vi "BuildAccessorFunctions.vi"(8 "error in (no error)":errorcluster, 11 "CS++Actor in":refnum<class "CS++Actor.lvclass">) -> (0 "error out":errorcluster, 3 "CS++Actor out":refnum<class "CS++Actor.lvclass">)   [LabVIEW 2016, in "CS++Actor.lvlib" / "CS++Actor.lvclass"]
uses:
  CS++Actor.lvclass
  CS++Actor.lvclass/CS++Actor.ctl
  <vilib>/Utility/traverseref.llb/TRef TravTarget.ctl
  <resource>/Framework/Providers/LVClassLibrary/NewAccessors/MemberVICreation.lvlib
  <vilib>/Utility/traverseref.llb/VI Scripting - Traverse.lvlib
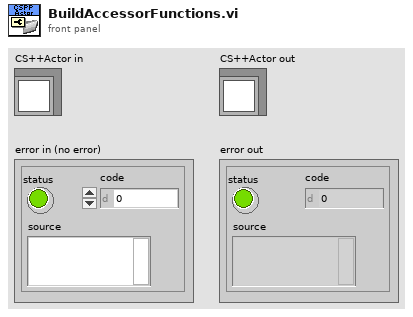
[diagram p1: front panel]
types:
  T1 = typedef "TRef TravTarget.ctl" = enum16{"FP", "BD", "Other"}
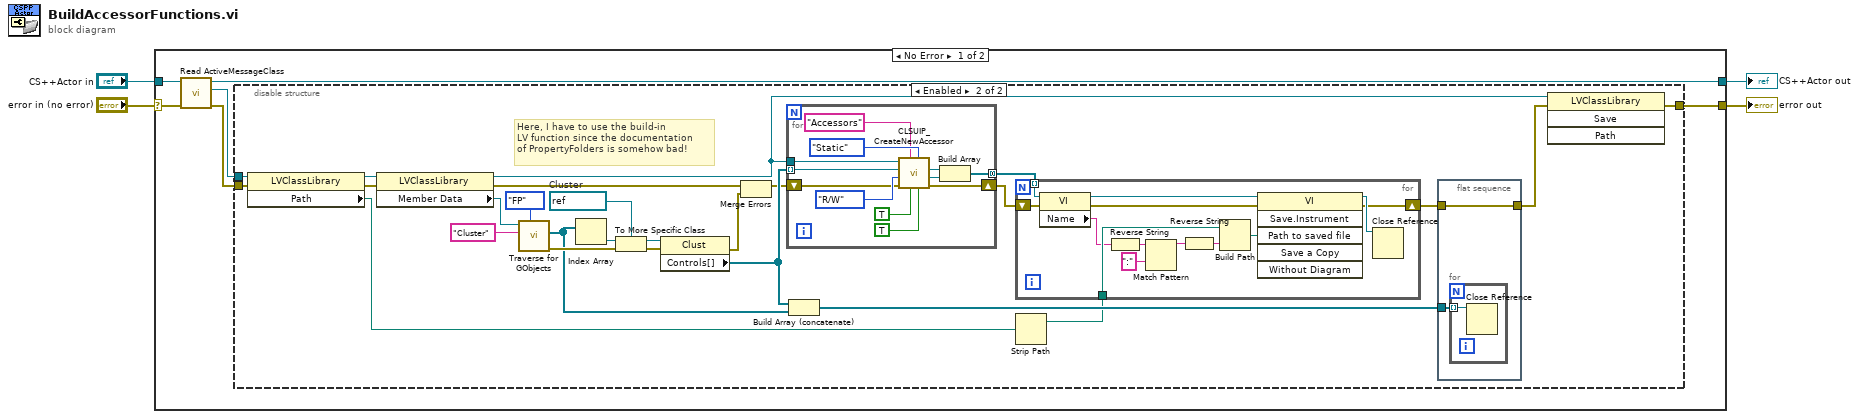
[diagram p0: block diagram]
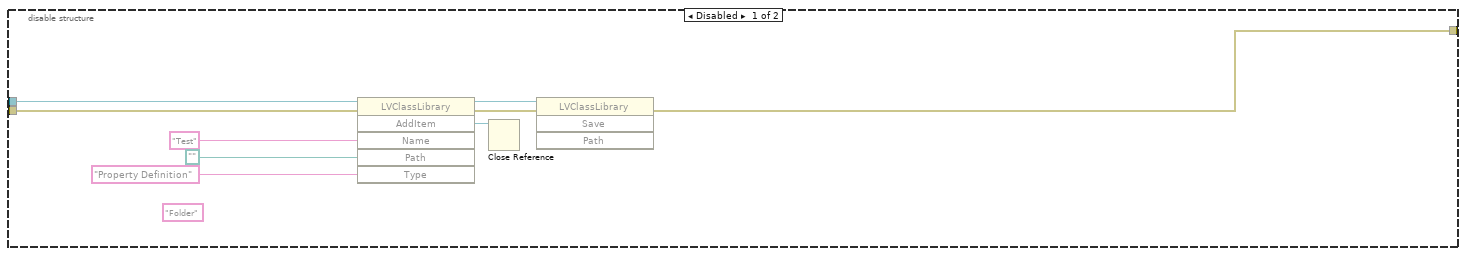
[diagram p2: hidden frame]
diagram:
  n1 = case shown="No Error" "error in (no error)" {
    selector: "error in (no error)" -> [w8 w75]
    tunnel: [w5 w75] -> w3
    tunnel: [w9 w74] -> w1
    tunnel: "CS++Actor in" -> [w10 w74]
    frame No Error {
      n2 = call "Read ActiveMessageClass.vi"("error in (no error)"=w8, "CS++Actor in"=w10) -> ("error out"=w6:errorcluster, "ActiveMessageClass"=w7:refnum<vi>, "CS++Actor out"=w9:refnum<class "CS++Actor.lvclass">)  [unwired: 7 in]
      n3 = disable-structure shown="Enabled" {
        disable-tunnel: w7 -> [w19 w29]
        disable-tunnel: w6 -> [w18 w27]
        disable-tunnel: [w12 w35] -> w5
        frame Disabled {
          (unwired) "Folder" ("Type")
          n4 = invoke class="LVClassLibrary" method="AddItem"(reference=w19, error in=w18, "Name"="Test" ("Type"), "Path"=path "", "Type"="Property Definition") -> (reference out=w14:refnum<vi>, error out=w13:errorcluster, "AddItem"=w15:refnum<vi>)  [unwired: 1 in, 3 out]
          n5 = Close Reference(reference=w15) -> ()  [unwired: 1 in, 1 out]
          n6 = invoke class="LVClassLibrary" method="Save"(reference=w14, error in=w13) -> (error out=w12:errorcluster)  [unwired: 2 in, 3 out]
        }
        frame Enabled {
          w42 = refnum<vi> refnum  # Cluster
          # "Here, I have to use the build-in\nLV function since the documentation\nof PropertyFolders is somehow bad!"
          n7 = property class="LVClassLibrary"(reference=w29, error in=w27) -> (reference out=w28:refnum<vi>, error out=w26:errorcluster, "Path"=w25:path)
          n8 = property class="LVClassLibrary"(reference=w28, error in=w26) -> (reference out=w33:refnum<vi>, error out=w22:errorcluster, "Member Data"=w38:refnum<vi>)
          n9 = call <vilib>:"Traverse for GObjects.vi"("Traverse Target"=TRef_TravTarget."FP", "Class Name"="Cluster" ("name/order"), "VI Refnum"=w38) -> ("error out"=w41:errorcluster, "References"=w36:refnum<vi>[])  [unwired: 5 in, 2 out]
          n10 = Index Array(array=w36) -> (element=w43:refnum<vi>)  [unwired: 1 in]
          n11 = To More Specific Class(target class=w42, reference=w43, error in=w41) -> (specific class reference=w39:refnum<vi>, error out=w40:errorcluster)
          n12 = property class="Clust"(reference=w39, error in=w40) -> (error out=w21:errorcluster, "Controls[]"=w23:refnum<vi>[])  [unwired: 1 out]
          n13 = Merge Errors(w22, w21) -> (w20:errorcluster)
          n14 = for {
            tunnel: w23 -> [w54] mode=indexing
            tunnel: w33 -> [w53]
            tunnel: [w50] -> w32 mode=concatenating
            shift-right: [w49] -> w31
            shift-left: w20 -> [w55]
            n15 = call <resource>:"CLSUIP_CreateNewAccessor.vi"("Make available through Property Nodes"=TRUE, "VI Type"=enum32{"Dynamic", "Static"}."Static", "Include error terminals"=TRUE, "Virtual Folder Name"="Accessors", "error in (no error)"=w55, "Access UI"=enum16{"Read", "Write", "R/W"}."R/W", "PDC Item Refnum"=w54, "LVClassLibrary Ref"=w53) -> ("error out"=w49:errorcluster, "Write VI"=w51:refnum<vi>, "Read VI"=w52:refnum<vi>)  [unwired: 1 in]
            n16 = Build Array(w52, w51) -> (w50:refnum<vi>[])
          }
          n17 = Build Array (concatenate)(w23, w36) -> (w37:refnum<vi>[])
          n18 = Strip Path(path=w25) -> (stripped path=w24:path)  [unwired: 1 out]
          n19 = for {
            tunnel: w32 -> [w71] mode=indexing
            shift-right: [w72] -> w30
            shift-left: w31 -> [w69]
            tunnel: w24 -> [w66]
            n20 = property class="VI"(reference=w71, error in=w69) -> (reference out=w70:refnum<vi>, error out=w68:errorcluster, "Name"=w65:string)
            n21 = Reverse String(1:w65) -> (0:w63:string)
            n22 = Match Pattern(string=w63, regular expression=":") -> (before substring=w62:string)  [unwired: 1 in, 3 out]
            n23 = Reverse String(1:w62) -> (0:w64:string)
            n24 = Build Path(base path=w66, name or relative path=w64) -> (appended path=w67:path)
            n25 = invoke class="VI" method="Save.Instrument"(reference=w70, error in=w68, "Path to saved file"=w67) -> (reference out=w73:refnum<vi>, error out=w72:errorcluster)  [unwired: 3 in, 4 out]
            n26 = Close Reference(reference=w73) -> ()  [unwired: 1 in, 1 out]
          }
          n27 = flat-sequence {
            tunnel: [w47] -> w34
            tunnel: w30 -> [w47]
            tunnel: w37 -> [w46]
            frame #0 {
              n28 = for {
                tunnel: w46 -> [w48] mode=indexing
                n29 = Close Reference(reference=w48) -> ()  [unwired: 1 in, 1 out]
              }
            }
          }
          n30 = invoke class="LVClassLibrary" method="Save"(reference=w33, error in=w34) -> (error out=w35:errorcluster)  [unwired: 2 in, 3 out]
        }
      }
    }
    frame Error {
    }
  }
  "error out" <- w3
  "CS++Actor out" <- w1
